vi "SetDriveMotorOutputsAuto.vi"(1 "RightMotorOutput":dbl, 2 "LeftMotorOutput":dbl) -> ()   [LabVIEW 2015]
uses:
  <vilib>/Rock Robotics/WPI/DriverStation/WPI_DriverStationRobotMode2.ctl
  Utilities/VisionGlobals.vi
  Utilities/GeneralGlobals.vi
panel:
  out "AutoTargetEnabled?":bool
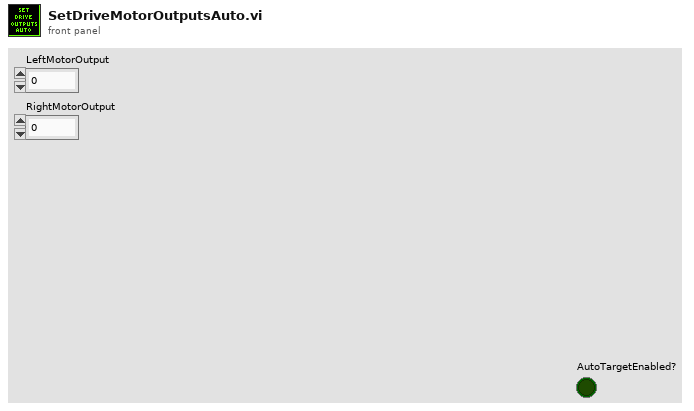
[diagram p1: front panel]
types:
  T1 = typedef "WPI_DriverStationRobotMode2.ctl" = enum16{"Autonomous Disabled", "Autonomous Enabled", "Teleop Disabled", "Teleop Enabled", "Disconnected", "Finish", "Test Disabled", "Test Enabled", "Emergency Stopped"}
  T2 = typedef "WPI_MotorControlDeviceRef.ctl" = cluster{"DeviceStatus":errorcluster, "Type":T3, "PWM":cluster{"PWM Channel":T4, "DeadBand":T5}, "CAN":cluster{"Device Number":u8, "Control Mode":T6, "Semaphore":T7, "Max Vout":dbl, "TalonSRX Control Mode":T8}, "Invert":bool}
  T3 = typedef "WPI_MotorControlType.ctl" = enum16{"PWM", "CAN", "CANTalonSRX"}
  T4 = typedef "FPGA_DIOPWMChannel.ctl" = enum8{"PWM 0", "PWM 1", "PWM 2", "PWM 3", "PWM 4", "PWM 5", "PWM 6", "PWM 7", "PWM 8", "PWM 9", "PWM MXP 0", "PWM MXP 1", "PWM MXP 2", "PWM MXP 3", "PWM MXP 4", "PWM MXP 5", "PWM MXP 6", "PWM MXP 7", "PWM MXP 8", "PWM MXP 9", "Invalid"}
  T5 = typedef "WPI_PWMDeadband.ctl" = cluster{"Name":string, "maxPositivePwm":i32, "minPositivePwm":i32, "centerPwm":i32, "maxNegativePwm":i32, "minNegativePwm":i32, "angularRange":u16}
  T6 = typedef "WPI_CANJaguar_ControlMode.ctl" = enum8{"Percent VBus", "Current", "Speed", "Position", "Voltage"}
  T7 = typedef "Semaphore RefNum" = refnum<k1>
  T8 = typedef "WPI_CANTalonSRX_APIControlMode.ctl" = enum8{"Percent VBus", "Speed", "Position", "Slave", "Unchanged / Invalid", "Voltage Compensation", "Current", "Motion Profile"}
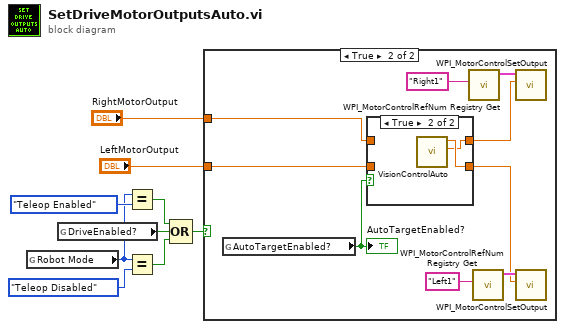
[diagram p0: block diagram]
diagram:
  n1 = global read "GeneralGlobals.vi" "Robot Mode"() -> (w1:T1)
  n2 = global read "VisionGlobals.vi" "DriveEnabled?"() -> (w5:bool)
  n3 = Equal?(x=w1, y=WPI_DriverStationRobotMode2."Teleop Enabled") -> (x = y?=w6:bool)
  n4 = Equal?(x=w1, y=WPI_DriverStationRobotMode2."Teleop Disabled") -> (x = y?=w2:bool)
  n5 = Compound Arithmetic op=OR(w6, w5, w2) -> (w4:bool)
  n6 = case shown="True" w4 {
    tunnel: "RightMotorOutput" -> [_ w10]
    tunnel: "LeftMotorOutput" -> [_ w11]
    frame False {
    }
    frame True {
      n7 = global read "VisionGlobals.vi" "AutoTargetEnabled?"() -> (w14:bool)
      "AutoTargetEnabled?" <- w14
      n8 = case shown="True" w14 {
        tunnel: [w20 w22] -> w13
        tunnel: [w19 w21] -> w12
        tunnel: w11 -> [w20 _]
        tunnel: w10 -> [w19 _]
        frame False {
        }
        frame True {
          n9 = call "VisionControlAuto.vi"() -> ("Right Drive"=w21:dbl, "Left Drive"=w22:dbl)  [unwired: 10 in]
        }
      }
      n10 = call <vilib>:"WPI_MotorControlRefNum Registry Get.vi"("refnum name"="Right1") -> ("MotorControlDevRef"=w18:T2)  [unwired: 9 in, 1 out]
      n11 = call <vilib>:"WPI_MotorControlRefNum Registry Get.vi"("refnum name"="Left1") -> ("MotorControlDevRef"=w16:T2)  [unwired: 9 in, 1 out]
      n12 = call <vilib>:"WPI_MotorControlSetOutput.vi"("Output"=w12, "MotorControlDevRef"=w18) -> ()  [unwired: 7 in, 3 out]
      n13 = call <vilib>:"WPI_MotorControlSetOutput.vi"("Output"=w13, "MotorControlDevRef"=w16) -> ()  [unwired: 7 in, 3 out]
    }
  }
